vi "schmit trigger not correct.vi"() -> ()   [LabVIEW 2016]
panel:
  out "Graph":dynamicdata(graph)
  out "Result  Graph":dynamicdata(graph)
  in  "LTP":dbl(slide) caption="Constant Value to Compare Against" scale=-1.0..1.0
  in  "UTP":dbl(slide) caption="Constant Value to Compare Against" scale=-1.0..1.0
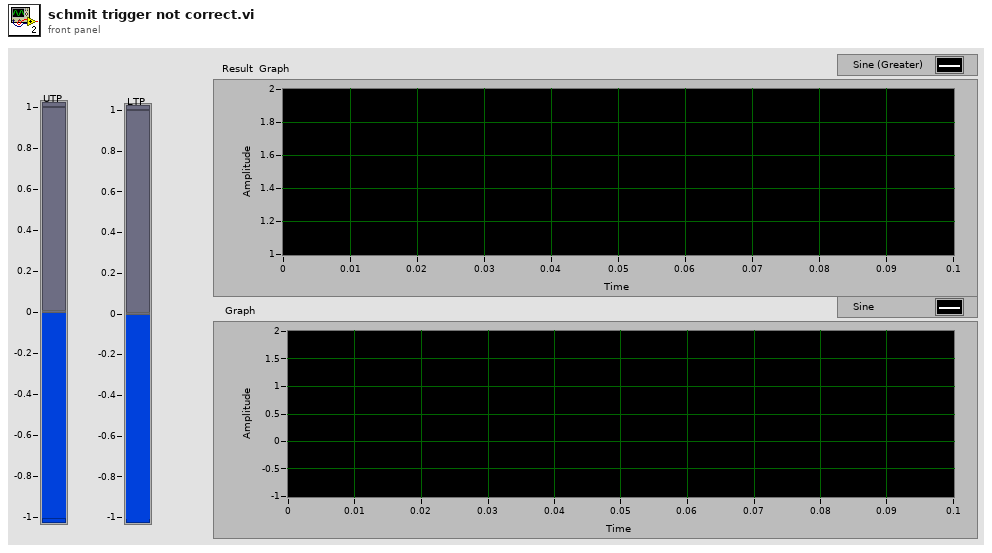
[diagram p1: front panel]
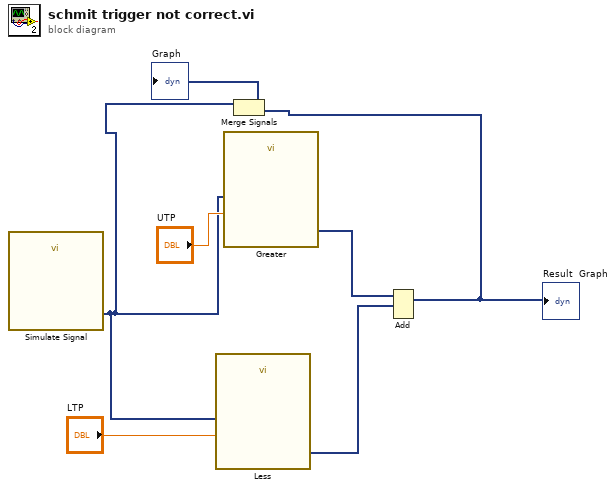
[diagram p0: block diagram]
diagram:
  n1 = call "Simulate Signal"() -> ("Sine"=w3:dynamicdata)  [unwired: 14 in, 1 out]
  n2 = call "Less"("Constant Value to Compare Against"="LTP", "Operand 1"=w3) -> ("Result"=w4:dynamicdata)  [unwired: 8 in, 1 out]
  n3 = call "Greater"("Constant Value to Compare Against"="UTP", "Operand 1"=w3) -> ("Result"=w5:dynamicdata)  [unwired: 8 in, 1 out]
  n4 = Add(1:w4, 2:w5) -> (0:w1:dynamicdata)  [unwired: 1 in, 1 out]
  "Result  Graph" <- w1
  n5 = Merge Signals(w3, w1) -> (→"Graph":dynamicdata)
